vi "ADC-NEW.vi"(0 "Analog_Data(V)":dbl=0.0001 min=-15.0 max=30.0 step=0.01, 5 "Voltage_Range(V)":dbl=1.0 min=1e-06 max=30.0 step=0.01, 7 "Resolution (bits)":i32=1 min=1 max=128, 11 "Stop":bool) -> (4 "Digital_Code":i64)   [LabVIEW 2021]
doc: "This VI converts analog value into Digital value."
panel:
  # "ADC"
  # "NOTE:\n This ADC system converts -V to +V and represent the respective Digital code from -(2^(n-1)-1) to (2^(n-1)).\n\nWhere n represent the Resolution (converted for which type of system, eg 8bit, 16bit, 32bit or 64bit systems)"
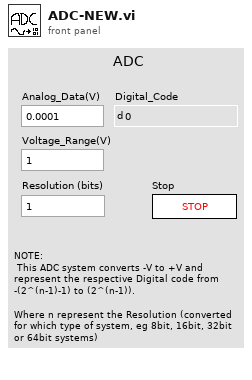
[diagram p1: front panel]
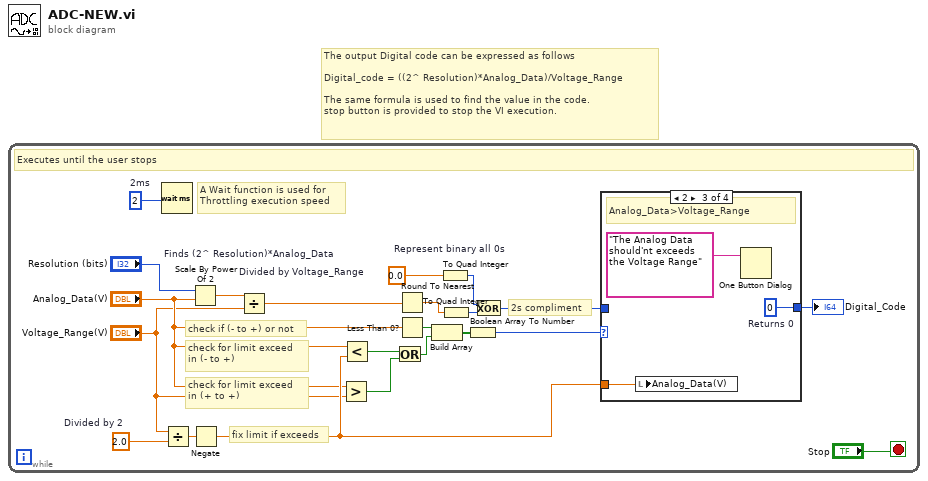
[diagram p0: block diagram]
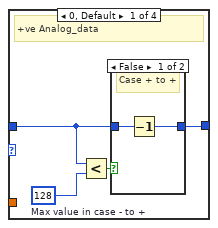
[diagram p2: hidden frame]
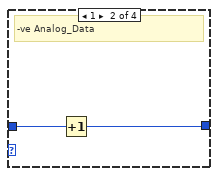
[diagram p4: hidden frame]
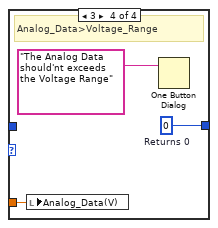
[diagram p5: hidden frame]
diagram:
  # "The output Digital code can be expressed as follows\n\nDigital_code = ((2^ Resolution)*Analog_Data)/Voltage_Range\n\nThe same formula is used to find the value in the code.\nstop button is provided to stop the VI execution."
  n1 = while {
    stop <- "Stop" stop-if-true
    w14 = 2.0  # Divided by 2
    w17 = 0.0  # Represent binary all 0s
    w22 = u32 2  # 2ms
    # "check for limit exceed \nin (+ to +)"
    # "check for limit exceed \nin (- to +)"
    # "fix limit if exceeds"
    # "check if (- to +) or not"
    # "2s compliment"
    # "A Wait function is used for \nThrottling execution speed"
    # "Executes until the user stops"
    n2 = Wait (ms)(milliseconds to wait=w22) -> ()  [unwired: 1 out]
    n3 = Divide(x="Voltage_Range(V)", y=w14) -> (x/y=w9:dbl)
    n4 = Scale By Power Of 2 "Finds (2^ Resolution)*Analog_Data"(n="Resolution (bits)", x="Analog_Data(V)") -> (x*2^n=w18:dbl)
    n5 = Negate(x=w9) -> (-x=w5:dbl)
    n6 = Divide "Divided by Voltage_Range"(x=w18, y="Voltage_Range(V)") -> (x/y=w19:dbl)
    n7 = Greater?(x="Analog_Data(V)", y="Voltage_Range(V)") -> (0:w1:bool)
    n8 = Less?(x="Analog_Data(V)", y=w5) -> (x < y?=w6:bool)
    n9 = Or(x=w6, y=w1) -> (x .or. y?=w2:bool)
    n10 = Round To Nearest(number=w19) -> (nearest integer value=w20:dbl)
    n11 = Less Than 0?(x="Analog_Data(V)") -> (x < 0?=w13:bool)
    n12 = Build Array(w13, w2) -> (w12:bool[])
    n13 = To Quad Integer(1:w17) -> (0:w8:i64)
    n14 = To Quad Integer(1:w20) -> (0:w7:i64)
    n15 = Boolean Array To Number(Boolean array=w12) -> (number=w11:u32)
    n16 = Exclusive Or(1:w7, 2:w8) -> (0:w15:i64)
    n17 = case shown="2" w11 {
      tunnel: w15 -> [w24 w31 _ _]
      tunnel: w5 -> [_ _ w32 w36]
      tunnel: [w26 w30 w33 w35] -> w10
      frame 0, Default {
        w23 = i64 128  # Max value in case - to +
        # "+ve Analog_data"
        n18 = Less?(x=w24, y=w23) -> (x < y?=w25:bool)
        n19 = case shown="False" w25 {
          tunnel: [w27 w29] -> w26
          tunnel: w24 -> [w28 w29]
          frame False {
            # "Case + to +"
            n20 = Decrement(x=w28) -> (x-1=w27:i64)
          }
          frame True {
            # "Case - to+"
          }
        }
      }
      frame 1 {
        # "-ve Analog_Data"
        n21 = Increment(x=w31) -> (x+1=w30:i64)
      }
      frame 2 {
        w33 = i64 0  # Returns 0
        # "Analog_Data>Voltage_Range"
        n22 = local write "Analog_Data(V)"(w32) -> ()
        n23 = One Button Dialog(message="The Analog Data should'nt exceeds the Voltage Range") -> ()  [unwired: 1 in, 1 out]
      }
      frame 3 {
        w35 = i64 0  # Returns 0
        # "Analog_Data>Voltage_Range"
        n24 = local write "Analog_Data(V)"(w36) -> ()
        n25 = One Button Dialog(message="The Analog Data should'nt exceeds the Voltage Range") -> ()  [unwired: 1 in, 1 out]
      }
    }
    "Digital_Code" <- w10
  }
